vi "Sort Plugins by Priority.vi"(8 "error in (no error)":errorcluster, 11 "Scheduler in":refnum<class "Scheduler.lvclass">) -> (0 "error out":errorcluster, 3 "Scheduler out":refnum<class "Scheduler.lvclass">)   [LabVIEW 2017, in "DSF Core.lvlib" / "Scheduler.lvclass"]
uses:
  Scheduler.lvclass
  Scheduler.lvclass/Scheduler.ctl
  Scheduler Plugin Bundle.lvclass
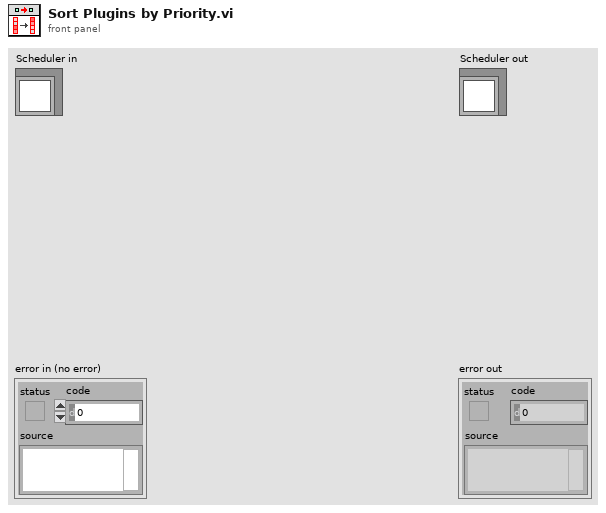
[diagram p1: front panel]
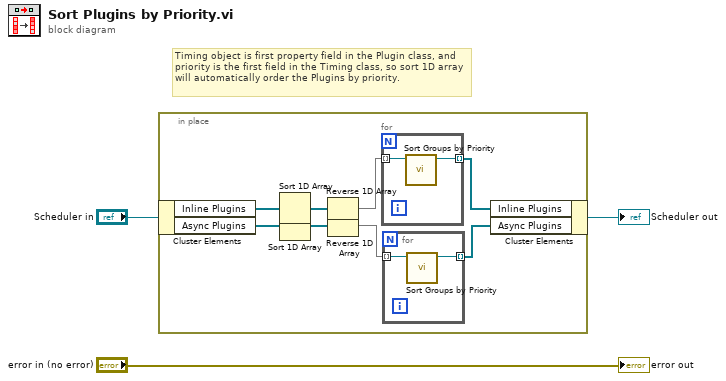
[diagram p0: block diagram]
diagram:
  # "Timing object is first property field in the Plugin class, and priority is the first field in the Timing class, so sort 1D array will automatically order the Plugins by priority."
  n1 = in-place {
    n2 = in-place-cluster #1("Scheduler in") -> ("Inline Plugins"=w11:refnum<class "Scheduler Plugin Bundle.lvclass">[], "Async Plugins"=w10:refnum<class "Scheduler Plugin Bundle.lvclass">[])
    n3 = Sort 1D Array(array=w11) -> (sorted array=w9:refnum<class "Scheduler Plugin Bundle.lvclass">[])
    n4 = Sort 1D Array(array=w10) -> (sorted array=w8:refnum<class "Scheduler Plugin Bundle.lvclass">[])
    n5 = Reverse 1D Array(array=w9) -> (reversed array=w7:refnum<class "Scheduler Plugin Bundle.lvclass">[])
    n6 = Reverse 1D Array(array=w8) -> (reversed array=w5:refnum<class "Scheduler Plugin Bundle.lvclass">[])
    n7 = for {
      tunnel: w7 -> [w15] mode=indexing
      tunnel: [w14] -> w6 mode=indexing
      n8 = call "Sort Groups by Priority.vi"("Scheduler Plugin Bundle in"=w15) -> ("Scheduler Plugin Bundle out"=w14:refnum<class "Scheduler Plugin Bundle.lvclass">)  [unwired: 9 in, 1 out]
    }
    n9 = for {
      tunnel: w5 -> [w13] mode=indexing
      tunnel: [w12] -> w4 mode=indexing
      n10 = call "Sort Groups by Priority.vi"("Scheduler Plugin Bundle in"=w13) -> ("Scheduler Plugin Bundle out"=w12:refnum<class "Scheduler Plugin Bundle.lvclass">)  [unwired: 9 in, 1 out]
    }
    n11 = in-place-cluster #1("Inline Plugins"=w6, "Async Plugins"=w4) -> (→"Scheduler out":refnum<class "Scheduler.lvclass">)
  }
  "error out" <- "error in (no error)"
